vi "PWM Configuration to Channel Settings.vi"(6 "PWM":T1 {"PWM Channels"."PWM frequency" items=["1 Hz", "50 Hz", "250 Hz", "500 Hz", "1 kHz", "5 kHz", "10 kHz", "20 kHz"]}, 8 "error in":errorcluster, 9 "default values":dbl[](array[numeric]), 10 "names":string[](array[string]), 11 "Mode in":refnum<class "Mode.lvclass">) -> (0 "error out":errorcluster, 2 "channel settings":T2[](array[typedef]), 3 "Mode out":refnum<class "Mode.lvclass">)   [LabVIEW 2017, in "Scan Engine Scripting.lvlib" / "Mode.lvclass"]
uses:
  Mode.lvclass
  Controls/pwm channel settings.ctl
  Channel Classes/PWM Output Channel/Frequency.ctl
  Channel Classes/PWM Output Channel/PWM Output Channel.lvclass
  Scan Engine Scripting.lvlib
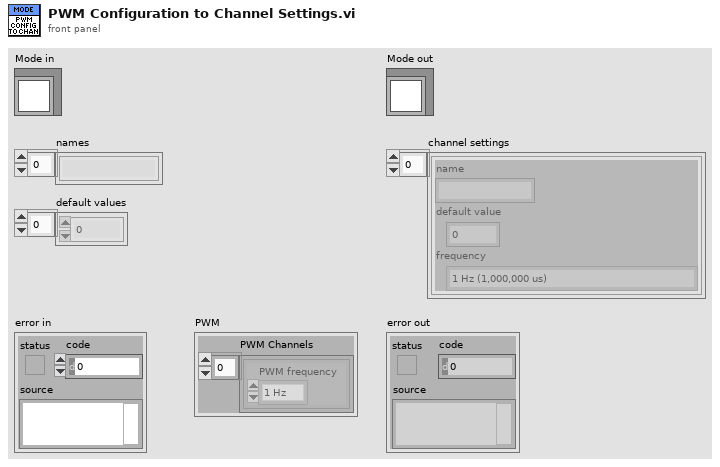
[diagram p1: front panel]
types:
  T1 = cluster{"PWM Channels":cluster{"PWM frequency":u32}[]}
  T2 = typedef "Scan Engine Scripting.lvlib/pwm channel settings.ctl" = cluster{"name":string, "default value":dbl, "frequency":T3}
  T3 = typedef "Scan Engine Scripting.lvlib/PWM Output Channel.lvclass/Frequency.ctl" = enum16{"1 Hz (1,000,000 us)", "50 Hz (20,000 us)", "250 Hz (4,000 us)", "500 Hz (2,000 us)", "1 kHz (1,000 us)", "5 kHz (200 us)", "10 kHz (100 us)", "20 kHz (50 us)"}
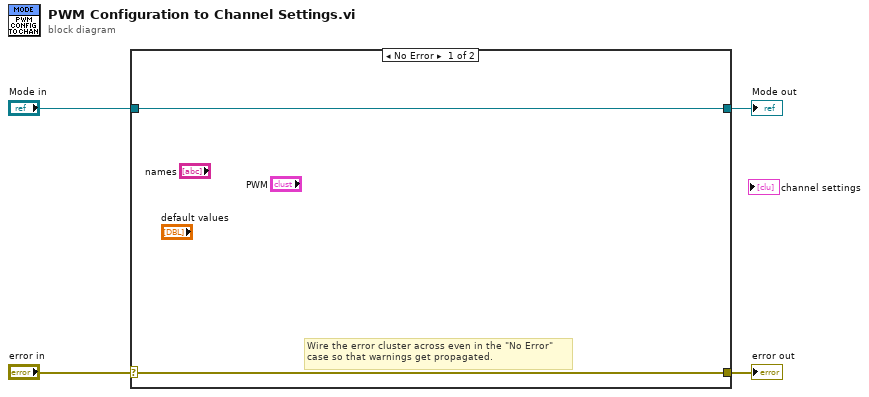
[diagram p0: block diagram]
diagram:
  n1 = case shown="No Error" "error in" {
    selector: "error in" -> [w5 w8]
    tunnel: [w5 w8] -> w3
    tunnel: [w6 w7] -> w1
    tunnel: "Mode in" -> [w6 w7]
    frame No Error {
      # "Wire the error cluster across even in the \"No Error\"\ncase so that warnings get propagated."
    }
    frame Error {
    }
  }
  "error out" <- w3
  "Mode out" <- w1
